vi "getSummaryState.vi"(11 "Model in":refnum<class "Model.lvclass">) -> (2 "SummaryStates":T1, 3 "Model out":refnum<class "Model.lvclass">)   [LabVIEW 2016, in "Model.lvclass"]
uses:
  Model.lvclass
  Types/SummaryStates.ctl
  Model.lvclass/Model.ctl
  Types/M1M3SupportTypes.lvlib
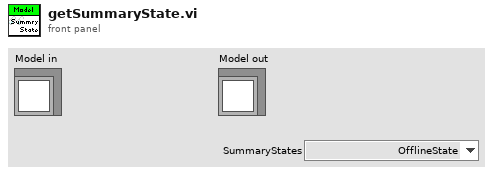
[diagram p1: front panel]
types:
  T1 = typedef "M1M3SupportTypes.lvlib/SummaryStates.ctl" = enum16{"OfflineState", "StandbyState", "DisabledState", "EnabledState", "FaultState"}
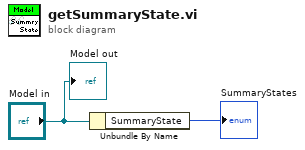
[diagram p0: block diagram]
diagram:
  n1 = Unbundle By Name("Model in") -> ("SummaryState"=→"SummaryStates":T1)
  "Model out" <- "Model in"
